vi "GetType.vi"(8 "error in (no error)":errorcluster, 11 "Configure StartVelocity Msg":refnum<class "Configure StartVelocity Msg.lvclass">) -> (0 "error out":errorcluster, 2 "Data Sample":variant, 3 "Configure StartVelocity Msg":refnum<class "Configure StartVelocity Msg.lvclass">)   [LabVIEW 2015, in "CS++Motor.lvlib" / "Configure StartVelocity Msg.lvclass"]
uses:
  Configure StartVelocity Msg.lvclass
  Configure StartVelocity Msg.lvclass/Configure StartVelocity Msg.ctl
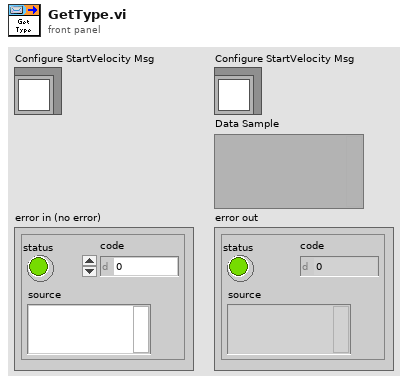
[diagram p1: front panel]
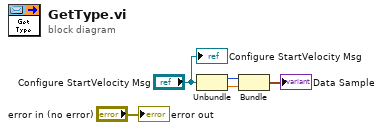
[diagram p0: block diagram]
diagram:
  n1 = Unbundle("Configure StartVelocity Msg") -> (w2:u8, w1:dbl)
  n2 = Bundle("AxisNumber"=w2, "StartVelocity"=w1) -> (→"Data Sample":cluster{"AxisNumber":u8, "StartVelocity":dbl})  [unwired: 1 in]
  "error out" <- "error in (no error)"
  "Configure StartVelocity Msg" <- "Configure StartVelocity Msg"
